vi "generateMove.vi"(1 "j":i32, 2 "i":i32) -> (0 "Array":i32[][](array[numeric]))   [LabVIEW 2024]
uses:
  globalVar.vi
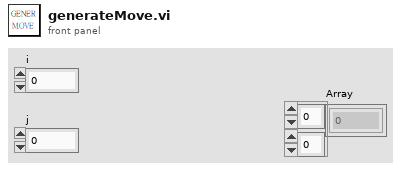
[diagram p1: front panel]
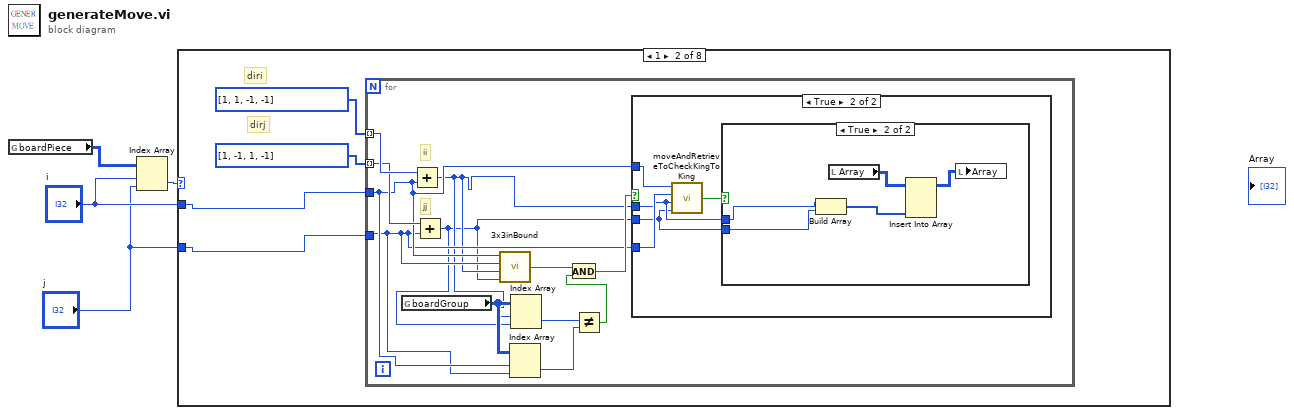
[diagram p0: block diagram]
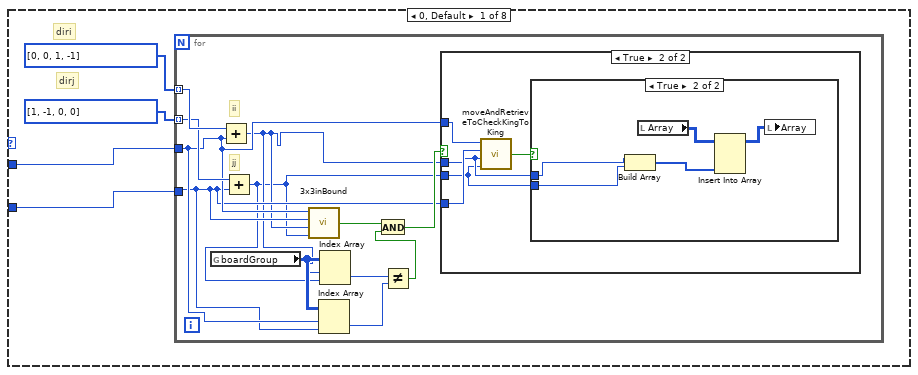
[diagram p2: hidden frame]
diagram:
  n1 = global read "globalVar.vi" "boardPiece"() -> (w4:i32[][])
  n2 = Index Array(array=w4, index (row)="i", index (col)="j") -> (element=w3:i32)
  n3 = case shown="1" w3 {
    tunnel: "i" -> [w8 w32 _ _ _ _ _ _]
    tunnel: "j" -> [w7 w31 _ _ _ _ _ _]
    frame 0, Default {
      # "dirj"
      # "diri"
      n4 = for {
        tunnel: w8 -> [w13]
        tunnel: w7 -> [w12]
        tunnel: i32[] [0, 0, 1, -1] -> [w20] mode=indexing
        tunnel: i32[] [1, -1, 0, 0] -> [w19] mode=indexing
        # "jj"
        # "ii"
        n5 = global read "globalVar.vi" "boardGroup"() -> (w17:i32[][])
        n6 = Add(x=w20, y=w13) -> (x+y=w11:i32)
        n7 = Add(x=w19, y=w12) -> (x+y=w10:i32)
        n8 = call "3x3inBound.vi"("jj"=w10, "ii"=w11, "j"=w12, "i"=w13) -> ("inBound"=w9:bool)
        n9 = Index Array(array=w17, index (row)=w13, index (col)=w12) -> (element=w16:i32)
        n10 = Index Array(array=w17, index (row)=w11, index (col)=w10) -> (element=w18:i32)
        n11 = Not Equal?(x=w18, y=w16) -> (x != y?=w15:bool)
        n12 = And(x=w9, y=w15) -> (x .and. y?=w14:bool)
        n13 = case shown="True" w14 {
          tunnel: w13 -> [_ w25]
          tunnel: w12 -> [_ w24]
          tunnel: w11 -> [_ w22]
          tunnel: w10 -> [_ w21]
          frame False {
          }
          frame True {
            n14 = call "moveAndRetrieveToCheckKingToKing.vi"("j2"=w21, "i2"=w22, "j1"=w24, "i1"=w25) -> ("isKingToKing"=w23:bool)
            n15 = case shown="True" w23 {
              tunnel: w22 -> [_ w30]
              tunnel: w21 -> [_ w29]
              frame False {
              }
              frame True {
                n16 = Build Array(w30, w29) -> (w28:i32[])
                n17 = local read "Array"() -> (w27:i32[][])
                n18 = Insert Into Array(array=w27, new element=w28) -> (w26:i32[][])  [unwired: 2 in]
                n19 = local write "Array"(w26) -> ()
              }
            }
          }
        }
      }
    }
    frame 1 {
      # "dirj"
      # "diri"
      n20 = for {
        tunnel: w32 -> [w39]
        tunnel: w31 -> [w38]
        tunnel: i32[] [1, 1, -1, -1] -> [w46] mode=indexing
        tunnel: i32[] [1, -1, 1, -1] -> [w45] mode=indexing
        # "jj"
        # "ii"
        n21 = global read "globalVar.vi" "boardGroup"() -> (w43:i32[][])
        n22 = Add(x=w46, y=w39) -> (x+y=w37:i32)
        n23 = Add(x=w45, y=w38) -> (x+y=w36:i32)
        n24 = call "3x3inBound.vi"("jj"=w36, "ii"=w37, "j"=w38, "i"=w39) -> ("inBound"=w35:bool)
        n25 = Index Array(array=w43, index (row)=w39, index (col)=w38) -> (element=w42:i32)
        n26 = Index Array(array=w43, index (row)=w37, index (col)=w36) -> (element=w44:i32)
        n27 = Not Equal?(x=w44, y=w42) -> (x != y?=w41:bool)
        n28 = And(x=w35, y=w41) -> (x .and. y?=w40:bool)
        n29 = case shown="True" w40 {
          tunnel: w39 -> [_ w51]
          tunnel: w38 -> [_ w50]
          tunnel: w37 -> [_ w48]
          tunnel: w36 -> [_ w47]
          frame False {
          }
          frame True {
            n30 = call "moveAndRetrieveToCheckKingToKing.vi"("j2"=w47, "i2"=w48, "j1"=w50, "i1"=w51) -> ("isKingToKing"=w49:bool)
            n31 = case shown="True" w49 {
              tunnel: w48 -> [_ w56]
              tunnel: w47 -> [_ w55]
              frame False {
              }
              frame True {
                n32 = Build Array(w56, w55) -> (w54:i32[])
                n33 = local read "Array"() -> (w53:i32[][])
                n34 = Insert Into Array(array=w53, new element=w54) -> (w52:i32[][])  [unwired: 2 in]
                n35 = local write "Array"(w52) -> ()
              }
            }
          }
        }
      }
    }
    frame 2 {
    }
    frame 3 {
    }
    frame 4 {
    }
    frame 5 {
    }
    frame 6 {
    }
    frame 7 {
    }
  }
